vi "CheckConnectedResponse.vi"(2 "message":T1, 5 "error in (no error)":errorcluster) -> (19 "error out":errorcluster)   [LabVIEW 2017, in "LabVIEW STOMP.lvlib" / "STOMP.lvclass"]
uses:
  STOMP.lvclass
  Typedefs/Type_ServerFrame.ctl
  Typedefs/Type_ServerFrameType.ctl
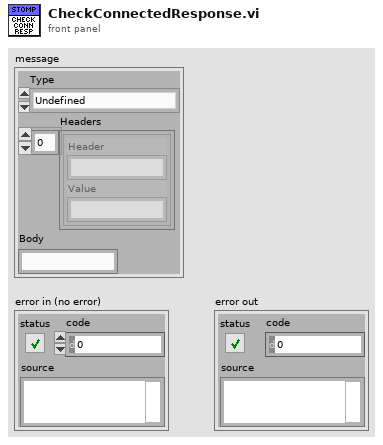
[diagram p1: front panel]
types:
  T1 = typedef "LabVIEW STOMP.lvlib/STOMP.lvclass/Type_ServerFrame.ctl" = cluster{"Type":T2, "Headers":cluster{"Header":string, "Value":string}[], "Body":string}
  T2 = typedef "LabVIEW STOMP.lvlib/STOMP.lvclass/Type_ServerFrameType.ctl" = enum16{"Undefined", "MESSAGE", "CONNECTED", "RECEIPT", "ERROR"}
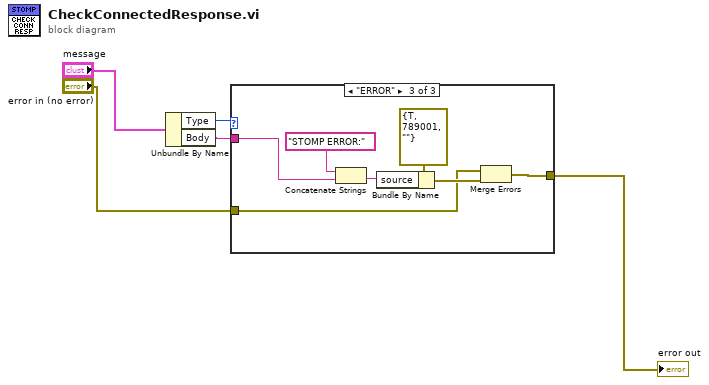
[diagram p0: block diagram]
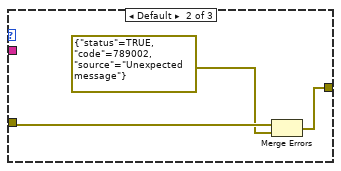
[diagram p3: hidden frame]
diagram:
  n1 = Unbundle By Name("message") -> ("Type"=w1:T2, "Body"=w2:string)
  n2 = case shown="\"ERROR\"" w1 {
    tunnel: w2 -> [_ _ w15]
    tunnel: "error in (no error)" -> [w6 w9 w13]
    tunnel: [w6 w7 w12] -> w3
    frame "CONNECTED" {
    }
    frame Default {
      n3 = Merge Errors(w9, errorcluster {"status"=TRUE, "code"=789002, "source"="Unexpected message"} ("error constant")) -> (w7:errorcluster)
    }
    frame "ERROR" {
      n4 = Concatenate Strings("STOMP ERROR:" ("string"), w15) -> (w11:string)
      n5 = Bundle By Name(cluster=errorcluster {"status"=TRUE, "code"=789001, "source"=""} ("error constant"), "source"=w11) -> (w14:errorcluster)
      n6 = Merge Errors(w13, w14) -> (w12:errorcluster)
    }
  }
  "error out" <- w3
